vi "gxml_GetArrayDim.vi"(7 "Empty Default Array?":bool, 8 "error in":errorcluster, 9 "offset (0)":i32, 10 "Flattened Data String":string, 11 "Dimensions":i32) -> (0 "error out":errorcluster, 1 "offset":i32, 3 "ArrayDimensions":i32[](array[numeric]), 5 "Element Count":i32)   [LabVIEW 2011, in "Third Party VIs.lvlib" / "GXML.lvlib"]
doc: "Uses the flattened data string (at position 'offset') to determine how many elements per dimension are in array."
uses:
  GXML.lvlib
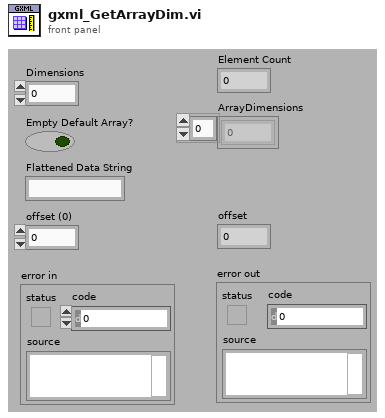
[diagram p1: front panel]
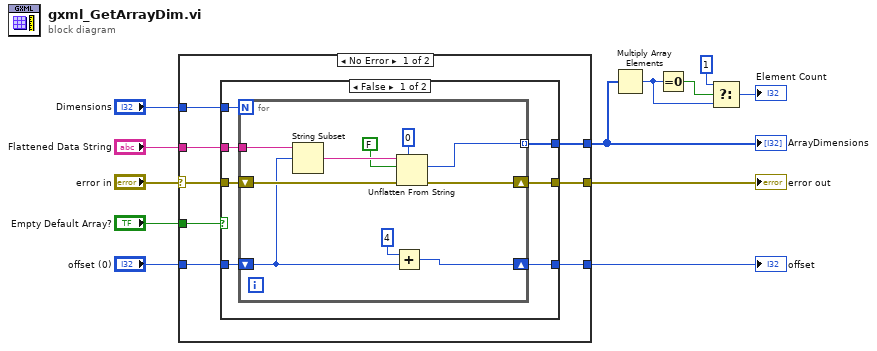
[diagram p0: block diagram]
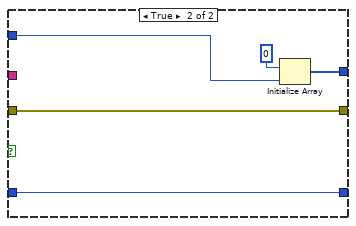
[diagram p2: hidden frame]
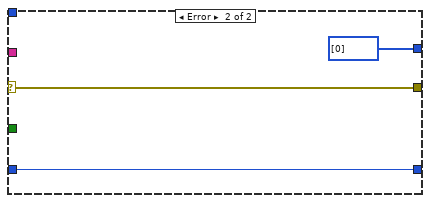
[diagram p3: hidden frame]
diagram:
  n1 = case shown="No Error" "error in" {
    selector: "error in" -> [w13 w45]
    tunnel: [w20 w45] -> w12
    tunnel: [w19 i32[] [0]] -> w2
    tunnel: "Dimensions" -> [w18 _]
    tunnel: [w17 w44] -> w10
    tunnel: "offset (0)" -> [w16 w44]
    tunnel: "Flattened Data String" -> [w15 _]
    tunnel: "Empty Default Array?" -> [w14 _]
    frame No Error {
      n2 = case shown="False" w14 {
        tunnel: [w27 w42] -> w20
        tunnel: [w26 w38] -> w19
        tunnel: w18 -> [w25 w40]
        tunnel: w13 -> [w24 w42]
        tunnel: [w23 w41] -> w17
        tunnel: w16 -> [w22 w41]
        tunnel: w15 -> [w21 _]
        frame False {
          n3 = for {
            N: w25 -> [_]
            tunnel: w21 -> [w37]
            shift-right: [w33] -> w23
            shift-left: w22 -> [w32]
            tunnel: [w34] -> w26 mode=indexing
            shift-right: [w35] -> w27
            shift-left: w24 -> [w36]
            n4 = String Subset(string=w37, offset (0)=w32) -> (substring=w31:string)  [unwired: 1 in]
            n5 = Add(x=4, y=w32) -> (x+y=w33:i32)
            n6 = Unflatten From String(type=0 ("number"), binary string=w31, data includes array or string size? (T)=FALSE, error in (no error)=w36) -> (value=w34:i32, error out=w35:errorcluster)  [unwired: 1 in, 1 out]
          }
        }
        frame True {
          n7 = Initialize Array(0, w40) -> (w38:i32[])
        }
      }
    }
    frame Error {
    }
  }
  "error out" <- w12
  "ArrayDimensions" <- w2
  "offset" <- w10
  n8 = Multiply Array Elements(1:w2) -> (0:w4:i32)
  n9 = Equal To 0?(x=w4) -> (x = 0?=w5:bool)
  n10 = Select(t=1, s=w5, f=w4) -> (s? t:f=→"Element Count":i32)
